vi "Add enum Type to JSON Schema.vi"(8 "error in (no error)":errorcluster, 11 "JSON Schema in":string) -> (0 "error out":errorcluster, 3 "JSON Schema out":string)   [LabVIEW 2019, in "JSON-Schema.lvlib"]
uses:
  JSON-Schema.lvlib
  <vilib>/JDP Science/JSONtext/Next JSON Value.vi
  <vilib>/JDP Science/JSONtext/String Subset.vi
  <vilib>/JDP Science/JSONtext/Parsing/Advance past next JSON Value (inlined COPY).vi
  <vilib>/JDP Science/JSONtext/Parsing/Advance past whitespace.vi
  <vilib>/JDP Science/JSONtext/Parsing/Advance past String.vi
  <vilib>/JDP Science/JSONtext/Parsing/Advance past Number.vi
  <vilib>/JDP Science/JSONtext/Parsing/Advance past Line Ending.vi
  <vilib>/JDP Science/JSONtext/Parsing/Parse Full Path or Item Name.vi
  <vilib>/JDP Science/JSONtext/Parsing/Advance past Array.vi
  <vilib>/JDP Science/JSONtext/Parsing/Advance past Object.vi
  <vilib>/JDP Science/JSONtext/support/Error Cluster From Code.vi
  <vilib>/JDP Science/JSONtext/Offset/Find Item Locations by Path.vi
  <vilib>/JDP Science/JSONtext/JSONtext.lvlib
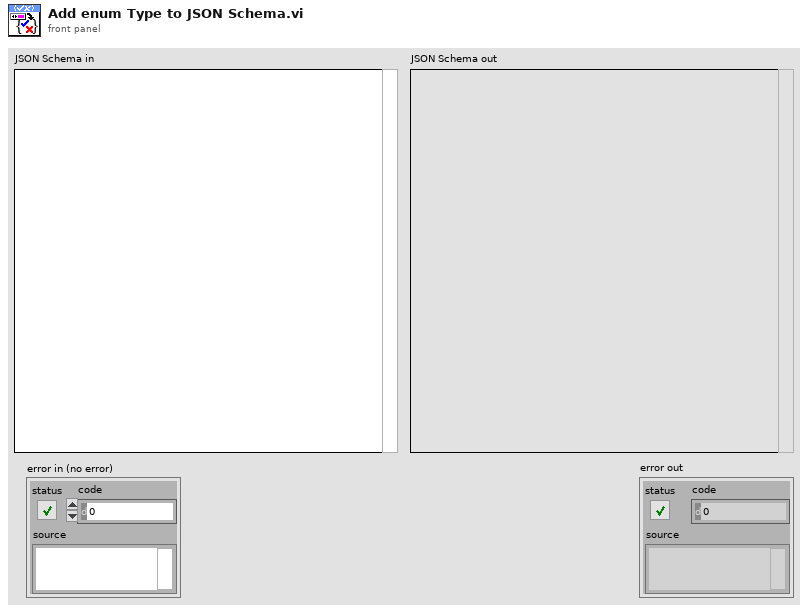
[diagram p1: front panel]
types:
  T1 = enum32{"Bad", "Idle", "Run top level", "Running"}
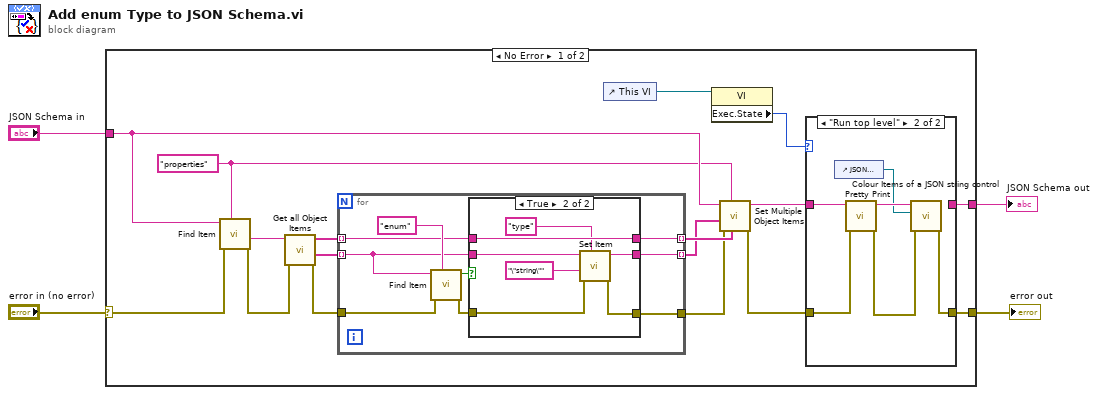
[diagram p0: block diagram]
diagram:
  n1 = case shown="No Error" "error in (no error)" {
    selector: "error in (no error)" -> [w11 w49]
    tunnel: "JSON Schema in" -> [w18 _]
    tunnel: [w8 w49] -> w2
    tunnel: [w5 _] -> w1
    frame No Error {
      w17 = "properties" ("$Path or Item Name")
      n2 = call <vilib>:"Find Item.vi"("$Path or Item Name"=w17, "error in (no error)"=w11, "JSON"=w18) -> ("error out"=w13:errorcluster, "<JSON>"=w12:string)  [unwired: 5 in, 2 out]
      n3 = call <vilib>:"Get all Object Items.vi"("error in (no error)"=w13, "JSON"=w12) -> ("error out"=w16:errorcluster, "<JSON>"=w14:string[], "Item Names"=w15:string[])  [unwired: 6 in, 1 out]
      n4 = for {
        tunnel: w14 -> [w36] mode=indexing
        tunnel: w15 -> [w35] mode=indexing
        tunnel: w16 -> [w37]
        tunnel: [w32] -> w19 mode=indexing
        tunnel: [w31] -> w20 mode=indexing
        tunnel: [w30] -> w10
        n5 = call <vilib>:"Find Item.vi"("$Path or Item Name"="enum", "error in (no error)"=w37, "JSON"=w36) -> ("error out"=w33:errorcluster, "Found"=w34:bool)  [unwired: 5 in, 2 out]
        n6 = case shown="True" w34 {
          tunnel: w36 -> [w41 w47]
          tunnel: w35 -> [w40 w44]
          tunnel: w33 -> [w39 w46]
          tunnel: [w41 w45] -> w32
          tunnel: [w40 w44] -> w31
          tunnel: [w39 w42] -> w30
          frame False {
          }
          frame True {
            n7 = call <vilib>:"Set Item.vi"("$Path or Item Name"="type", "error in (no error)"=w46, "JSON to Insert"="\"string\"" ("$Path or Item Name"), "JSON"=w47) -> ("error out"=w42:errorcluster, "<JSON>"=w45:string)  [unwired: 4 in, 1 out]
          }
        }
      }
      n8 = control-ref of="This VI"() -> (w7:refnum<vi>)
      n9 = property class="VI"(reference=w7) -> ("Exec.State"=w6:T1)  [unwired: 1 in, 2 out]
      n10 = call <vilib>:"Set Multiple Object Items.vi"("Item Names"=w20, "$Path or Item Name"=w17, "error in (no error)"=w10, "JSON Items"=w19, "JSON"=w18) -> ("error out"=w9:errorcluster, "<JSON>"=w21:string)  [unwired: 4 in]
      n11 = case shown="\"Run top level\"" w6 {
        tunnel: w21 -> [w22 w28]
        tunnel: w9 -> [w23 w27]
        tunnel: [w23 w25] -> w8
        tunnel: [w22 _] -> w5
        frame Default {
        }
        frame "Run top level" {
          n12 = control-ref of="JSON Schema out"() -> (w24:refnum<vi>)
          n13 = call <vilib>:"Pretty Print.vi"("error in (no error)"=w27, "JSON"=w28) -> ("error out"=w26:errorcluster, "<JSON>"=w29:string)  [unwired: 7 in, 1 out]
          n14 = call <vilib>:"Colour Items of a JSON string control.vi"("error in (no error)"=w26, "String Control"=w24, "JSON"=w29) -> ("error out"=w25:errorcluster)  [unwired: 8 in]
        }
      }
    }
    frame Error {
    }
  }
  "JSON Schema out" <- w1
  "error out" <- w2
